vi "Do.vi"(8 "error in (no error)":errorcluster, 10 "Actor in":refnum<class "Actor.lvclass">, 11 "Initiallize EMG Task Msg in":refnum<class "Initiallize EMG Task Msg.lvclass">) -> (0 "error out":errorcluster, 2 "Actor out":refnum<class "Actor.lvclass">)   [LabVIEW 2020, in "NI Force Task.lvlib" / "Initiallize EMG Task Msg.lvclass"]
doc: "(<B>Filename</B>: Actor Framework.lvlib:Message.lvclass:Do.vi)\n\nDefines what a message does when it is received by an actor. Generally, a message instructs an actor to invoke one of its methods. By default, this method does nothing. A child class must override it to define behavior. Create a child class by using the Actor Framework Message Maker dialog box."
uses:
  Initiallize EMG Task Msg.lvclass
  <vilib>/ActorFramework/Actor/Actor.lvclass
  NI Force Task/NI Force Task.lvclass
  C:/Program Files/National Instruments/LabVIEW 2020/vi.lib/ActorFramework/Actor/Actor.lvclass
  Initiallize EMG Task Msg.lvclass/Initiallize EMG Task Msg.ctl
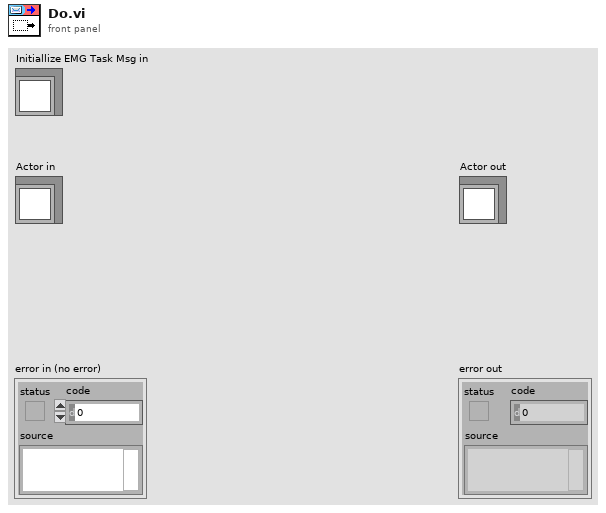
[diagram p1: front panel]
types:
  T1 = typedef "EMG channels df.ctl" = cluster{"EMG Master":bool, "EMGL1":tag, "EMGR1":tag, "EMGL2":tag, "EMGR2":tag, "EMGL3":tag, "EMGR3":tag, "EMGL4":tag, "EMGR4":tag, "EMGL5":tag, "EMGR5":tag, "EMGL6":tag, "EMGR6":tag, "EMGL7":tag, "EMGR7":tag, "EMGL8":tag, "EMGR8":tag}
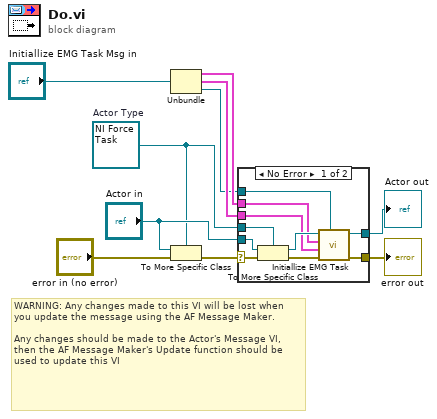
[diagram p0: block diagram]
diagram:
  w5 = refnum<class "NI Force Task.lvclass"> refnum  # Actor Type
  # "WARNING: Any changes made to this VI will be lost when you update the message using the AF Message Maker.\n\nAny changes should be made to the Actor's Message VI, then the AF Message Maker's Update function should be used to update this VI"
  n1 = Unbundle("Initiallize EMG Task Msg in") -> (w4:cluster{"Collect EMG?":bool, "EMG Rate":u16}, w3:T1, w2:refnum<k34>)
  n2 = To More Specific Class(target class=w5, reference="Actor in", error in="error in (no error)") -> (error out=w9:errorcluster)  [unwired: 1 out]
  n3 = case shown="No Error" w9 {
    selector: w9 -> [w20 w22]
    tunnel: [w15 w22] -> w8
    tunnel: [w14 w21] -> w7
    tunnel: "Actor in" -> [w19 w21]
    tunnel: w5 -> [w18 _]
    tunnel: w4 -> [w13 _]
    tunnel: w3 -> [w12 _]
    tunnel: w2 -> [w11 _]
    frame No Error {
      n4 = To More Specific Class ("Actor Cast")(target class=w18, reference=w19, error in=w20) -> (specific class reference=w17:refnum<class "NI Force Task.lvclass">, error out=w16:errorcluster)
      n5 = call "Initiallize EMG Task.vi"("TDMS File"=w11, "error in (no error)"=w16, "EMG Master Config"=w12, "EMG info"=w13, "NI Force Task in"=w17) -> ("error out"=w15:errorcluster, "NI Force Task out"=w14:refnum<class "NI Force Task.lvclass">)  [unwired: 5 in]
    }
    frame Error {
    }
  }
  "error out" <- w8
  "Actor out" <- w7
